vi "Write Data Access.vi"(8 "error in (no error)":errorcluster, 10 "Data Access":refnum<class "Data Access Engine.lvclass">, 11 "Process in":refnum<class "Process.lvclass">) -> (0 "error out":errorcluster, 3 "Process out":refnum<class "Process.lvclass">)   [LabVIEW 2027, in "VS Inline Async API.lvlib" / "Process.lvclass"]
uses:
  Process.lvclass
  _Data Access Engine/Data Access Engine/Data Access Engine.lvclass
  Process.lvclass/Process.ctl
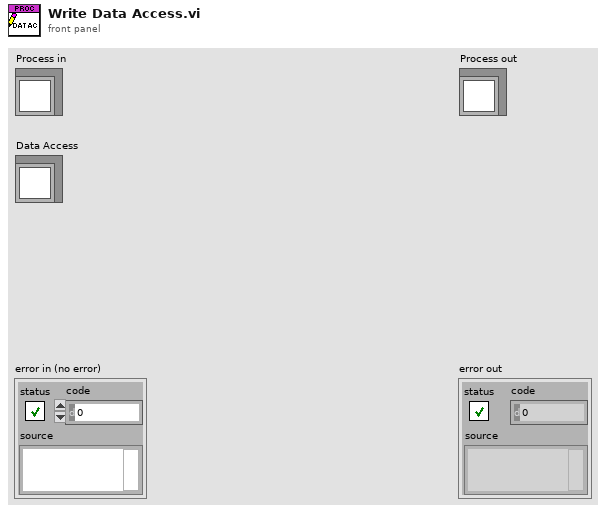
[diagram p1: front panel]
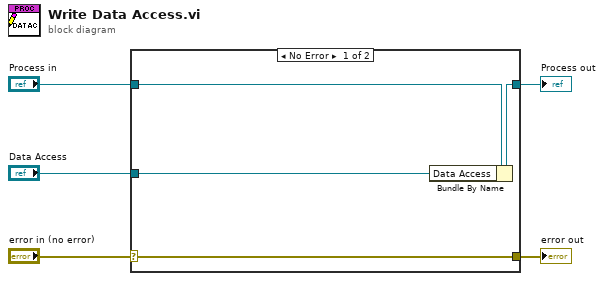
[diagram p0: block diagram]
diagram:
  n1 = case shown="No Error" "error in (no error)" {
    selector: "error in (no error)" -> [w9 w10]
    tunnel: [w9 w10] -> w4
    tunnel: [w7 w11] -> w2
    tunnel: "Process in" -> [w8 w11]
    tunnel: "Data Access" -> [w6 _]
    frame No Error {
      n2 = Bundle By Name(cluster=w8, "Data Access"=w6) -> (w7:refnum<class "Process.lvclass">)
    }
    frame Error {
    }
  }
  "error out" <- w4
  "Process out" <- w2
